vi "Inverse Kinematics.vi"(4 "Side":T2, 6 "Tolerance":dbl=0.1, 9 "Start":dbl[](array[numeric])=[0.0, -45.0, 0.0, 45.0, 0.0, 90.0, 0.0] format="%.3f", 10 "Goal-matrix":T1 format="%.3f", 11 "Label":string) -> (0 "Found":bool, 1 "Error":dbl, 2 "J":dbl[](array[numeric]) format="%.3f", 3 "Label":string)   [LabVIEW 2013]
uses:
  <vilib>/Analysis/Matrix/Datatypes/RealMatrix.ctl
  ROS/Code/SubVIs/BaxterSide.ctl
  <vilib>/Analysis/baseanly.llb/Real A x B.vi
  Fwd Kenimatics - array.vi
  <vilib>/Analysis/baseanly.llb/Real Inverse Matrix.vi
  Arm Globals.vi
  <vilib>/Analysis/NI_AALBase.lvlib
  <vilib>/Analysis/Matrix/NI_Matrix.lvlib
panel:
  in  "Joints":dbl[](array[numeric])=[0.0, 0.0, 0.0, 0.0, 0.0, -0.0, 0.0]
  out "Matrix":T1 format="%.3f"
  out "A x B":T1 format="%.3f"
  out "appended array":dbl[](array[numeric]) format="%.1f"
  out "Error History":dbl[](array[numeric])
  out "step":dbl format="%.6f"
  out "Count":i32
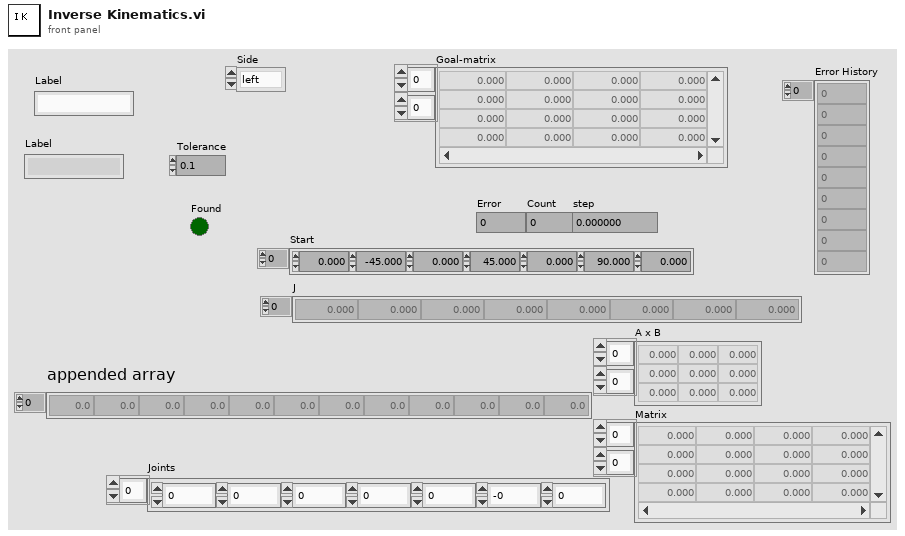
[diagram p1: front panel]
types:
  T1 = typedef "NI_Matrix.lvlib/RealMatrix.ctl" = dbl[][]
  T2 = typedef "BaxterSide.ctl" = enum16{"left", "right"}
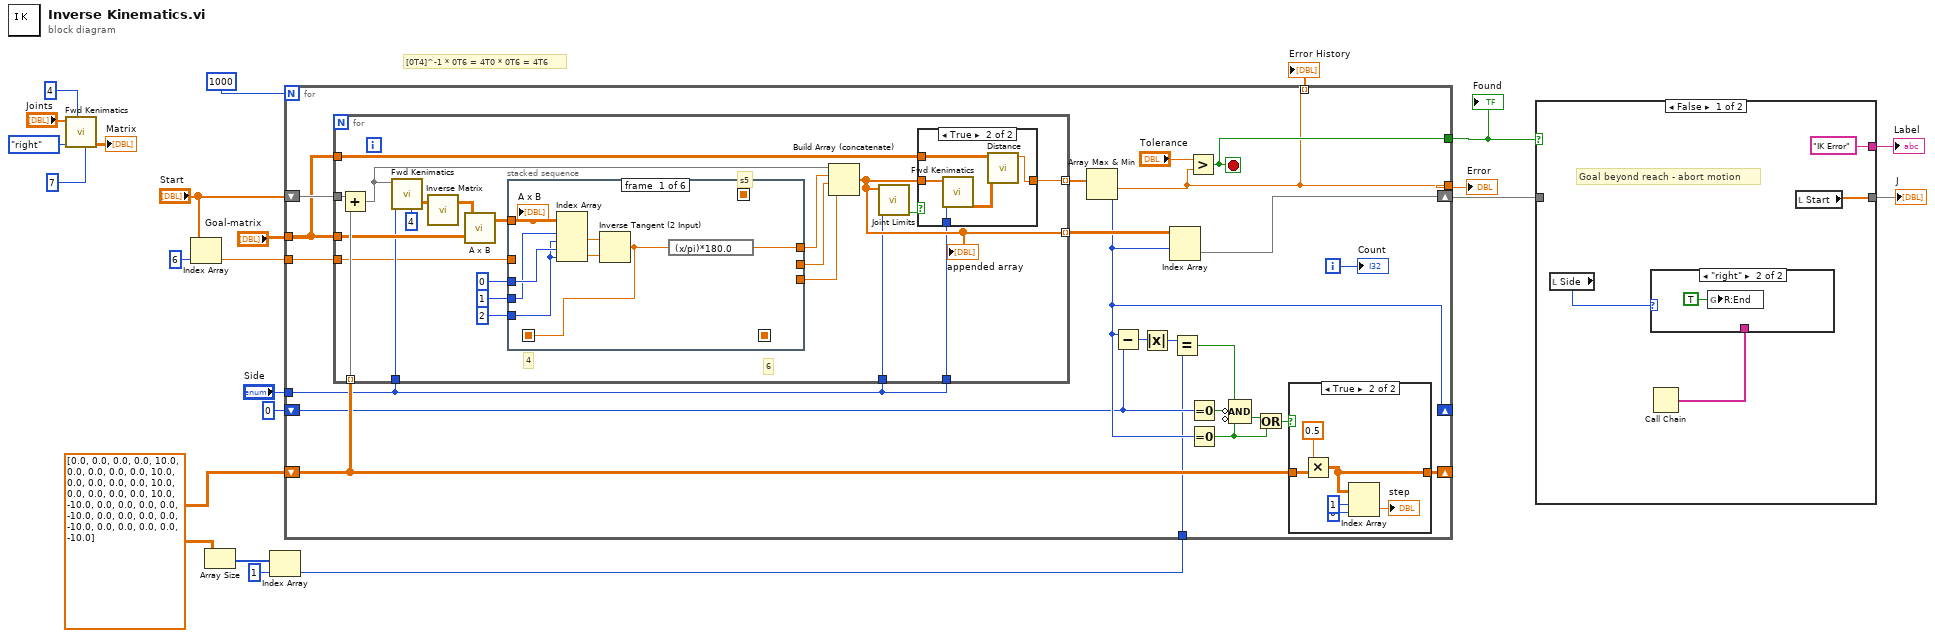
[diagram p0: block diagram]
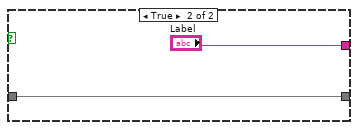
[diagram p3: hidden frame]
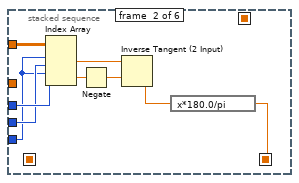
[diagram p5: hidden frame]
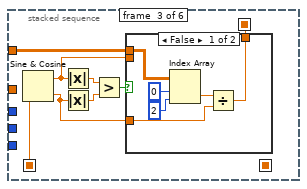
[diagram p6: hidden frame]
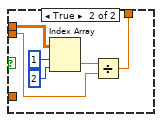
[diagram p7: hidden frame]
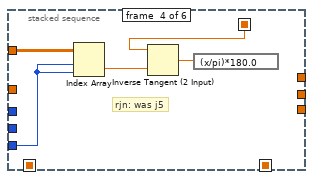
[diagram p8: hidden frame]
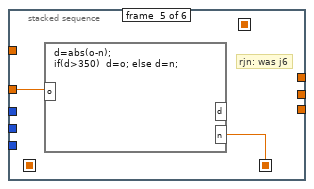
[diagram p9: hidden frame]
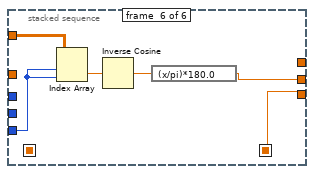
[diagram p10: hidden frame]
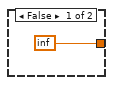
[diagram p11: hidden frame]
diagram:
  w16 = dbl[][] [[0.0, 0.0, 0.0, 0.0], [10.0, 0.0, 0.0, 0.0], [0.0, 10.0, 0.0, 0.0], [0.0, 0.0, 10.0, 0.0], [0.0, 0.0, 0.0, 10.0], [-10.0, 0.0, 0.0, 0.0], [0.0, -10.0, 0.0, 0.0], [0.0, 0.0, -10.0, 0.0], [0.0, 0.0, 0.0, -10.0]]
  # "[0T4]^-1 * 0T6 = 4T0 * 0T6 = 4T6"
  n1 = call-poly "Fwd Kenimatics.vi"("To"=7, "From"=4, "Side"=BaxterSide."right", "Joints"="Joints") -> ("Matrix"=→"Matrix":T1)  [unwired: 6 in, 1 out]
  n2 = Index Array(array="Start", index=6) -> (element=w9:dbl)
  n3 = Array Size(array=w16) -> (size(s)=w19:i32[])
  n4 = Index Array(array=w19, index=1) -> (element=w17:i32)
  n5 = for {
    N: 1000 -> [_]
    shift-right: [w43] -> w13
    shift-left: "Start" -> [w30]
    tunnel: [w24] -> w22
    shift-right: [w41] -> _
    shift-left: w16 -> [w40]
    shift-right: [w39] -> _
    shift-left: 0 -> [w32]
    tunnel: "Goal-matrix" -> [w26]
    tunnel: w17 -> [w29]
    tunnel: [w28] -> w8
    tunnel: "Side" -> [w25]
    tunnel: [w24] -> w14 mode=indexing
    tunnel: w9 -> [w23]
    i -> [w42]
    stop <- w28 stop-if-true
    n6 = for {
      tunnel: w40 -> [w70] mode=indexing
      tunnel: [w73] -> w45 mode=indexing
      tunnel: [w68] -> w44 mode=indexing
      tunnel: w30 -> [w71]
      tunnel: w26 -> [w69]
      tunnel: w26 -> [w60]
      tunnel: w25 -> [w56]
      tunnel: w25 -> [w55]
      tunnel: w25 -> [w54]
      tunnel: w23 -> [w53]
      # "6"
      # "s5"
      # "4"
      n7 = Add(x=w71, y=w70) -> (x+y=w57:dbl[])
      n8 = call-poly "Fwd Kenimatics.vi"("To"=4 ("# of Angles"), "Side"=w56, "Joints"=w57) -> ("Matrix"=w58:T1)  [unwired: 7 in, 1 out]
      n9 = call-poly <vilib>:"Inverse Matrix.vi"("Input Matrix"=w58) -> ("Inverse Matrix"=w67:T1)  [unwired: 1 in, 1 out]
      n10 = call-poly <vilib>:"A x B.vi"("B"=w69, "A"=w67) -> ("A x B"=w66:T1)  [unwired: 1 out]
      n11 = stacked-sequence {
        seq-local: [w78 _ _ _ _ _] -> [_ _ w99 _ _ _]
        seq-local: [_ _ w92 _ _ _] -> [_ _ _ w113 _ _]
        seq-local: [_ w83 _ _ _ _] -> [_ _ _ _ w118 w119]
        tunnel: [_ _ _ _ _ w119] -> w64
        tunnel: [w79 _ _ _ _ _] -> w72
        tunnel: w66 -> [w80 w90 w93 w116 _ w124]
        tunnel: [_ _ _ _ _ w120] -> w65
        tunnel: 0 ("index (col)") -> [w77 w86 _ _ _ _]
        tunnel: 1 ("index (row)") -> [w76 w85 _ _ _ _]
        tunnel: 2 ("index (row)") -> [w75 w84 _ w115 _ w123]
        tunnel: w53 -> [_ _ _ _ w117 _]
        frame #0 {
          n12 = Index Array(array=w80, index (row) #1=w76, index (col) #1=w75, index (row) #2=w77, index (col) #2=w75) -> (element #1=w81:dbl, element #2=w82:dbl)
          n13 = Inverse Tangent (2 Input)(1:w82, 2:w81) -> (0:w78:dbl)
          n14 = expression code="(x/pi)*180.0" ("radians to degrees")(w78) -> (w79:dbl)
          "A x B" <- w80
        }
        frame #1 {
          n15 = Index Array(array=w90, index (row) #1=w84, index (col) #1=w85, index (row) #2=w84, index (col) #2=w86) -> (element #1=w91:dbl, element #2=w89:dbl)
          n16 = Negate(x=w89) -> (-x=w88:dbl)
          n17 = Inverse Tangent (2 Input)(1:w88, 2:w91) -> (0:w87:dbl)
          n18 = expression code="x*180.0/pi" ("radians to degrees")(w87) -> (w83:dbl)
        }
        frame #2 {
          n19 = Sine & Cosine(0:w99) -> (1:w95:dbl, 2:w94:dbl)
          n20 = Absolute Value(x=w95) -> (abs(x)=w98:dbl)
          n21 = Absolute Value(x=w94) -> (abs(x)=w97:dbl)
          n22 = Greater?(x=w98, y=w97) -> (0:w96:bool)
          n23 = case shown="False" w96 {
            tunnel: w95 -> [_ w107]
            tunnel: w94 -> [w101 _]
            tunnel: w93 -> [w102 w111]
            tunnel: [w100 w106] -> w92
            frame False {
              n24 = Index Array(array=w102, index (row)=0, index (col)=2 ("disabled index (col)")) -> (element=w105:dbl)
              n25 = Divide(x=w105, y=w101) -> (x/y=w100:dbl)
            }
            frame True {
              n26 = Index Array(array=w111, index (row)=1, index (col)=2 ("disabled index (col)")) -> (element=w108:dbl)
              n27 = Divide(x=w108, y=w107) -> (x/y=w106:dbl)
            }
          }
        }
        frame #3 {
          # "rjn: was j5"
          n28 = Index Array(array=w116, index (row)=w115, index (col)=w115) -> (element=w114:dbl)
          n29 = Inverse Tangent (2 Input)(1:w114, 2:w113) -> (0:w112:dbl)
          n30 = expression code="(x/pi)*180.0" ("radians to degrees")(w112) -> ()  [unwired: 1 out]
        }
        frame #4 {
          # "rjn: was j6"
          n31 = formula code="d=abs(o-n);\nif(d>350)  d=o; else d=n;"("o"=w117, "n"=w118) -> ()  [unwired: 1 out]
        }
        frame #5 {
          n32 = Index Array(array=w124, index (row)=w123, index (col)=w123) -> (element=w122:dbl)
          n33 = Inverse Cosine(1:w122) -> (0:w121:dbl)
          n34 = expression code="(x/pi)*180.0" ("radians to degrees")(w121) -> (w120:dbl)
        }
      }
      n35 = Build Array (concatenate)(w57, w72, w65, w64) -> (w68:dbl[])
      "appended array" <- w68
      n36 = call "Joint Limits.vi"("Side"=w54, "Joints"=w68) -> ("In Range"=w74:bool)  [unwired: 9 in]
      n37 = case shown="True" w74 {
        tunnel: w68 -> [_ w130]
        tunnel: [inf w126] -> w73
        tunnel: w60 -> [_ w129]
        tunnel: w55 -> [_ w128]
        frame False {
        }
        frame True {
          n38 = call-poly "Fwd Kenimatics.vi"("Side"=w128, "Joints"=w130) -> ("Matrix"=w127:T1)  [unwired: 8 in, 1 out]
          n39 = call "Distance.vi"("Pose 2"=w127, "Pose 1"=w129) -> ("Distance"=w126:dbl)  [unwired: 9 in]
        }
      }
    }
    n40 = Array Max & Min(array=w45) -> (min value=w24:dbl, min index (indices)=w39:i32)  [unwired: 2 out]
    n41 = Subtract(x=w39, y=w32) -> (x-y=w38:i32)
    n42 = Absolute Value(x=w38) -> (abs(x)=w37:i32)
    n43 = Index Array(array=w44, index (row)=w39) -> (element=w43:dbl[])  [unwired: 1 in]
    n44 = Equal?(x=w37, y=w29) -> (x = y?=w34:bool)
    n45 = Greater?(x="Tolerance", y=w24) -> (0:w28:bool)
    n46 = Equal To 0?(x=w32) -> (x = 0?=w31:bool)
    n47 = Equal To 0?(x=w39) -> (x = 0?=w33:bool)
    n48 = Compound Arithmetic op=AND(w34, invert w31, invert w33) -> (w36:bool)
    n49 = Or(x=w36, y=w33) -> (x .or. y?=w35:bool)
    n50 = case shown="True" w35 {
      tunnel: w40 -> [w46 w52]
      tunnel: [w46 w50] -> w41
      frame False {
      }
      frame True {
        n51 = Multiply(x=0.5, y=w52) -> (x*y=w50:dbl[][])
        n52 = Index Array(array=w50, index (row)=1, index (col)=0 ("disabled index (col)")) -> (element=→"step":dbl)
      }
    }
    "Count" <- w42
  }
  "Error" <- w22
  "Found" <- w8
  "Error History" <- w14
  n53 = case shown="False" w8 {
    tunnel: w13 -> [_ w137]
    tunnel: [w134 w137] -> w7
    tunnel: ["IK Error" ("Label") "Label"] -> w6
    frame False {
      # "Goal beyond reach - abort motion"
      n54 = local read "Side"() -> (w132:T2)
      n55 = Call Chain() -> (call chain=w131:string[])
      n56 = case shown="\"right\"" w132 {
        tunnel: w131 -> [_ _]
        frame "left", Default {
        }
        frame "right" {
          n57 = global write "Arm Globals.vi" "R:End"(TRUE ("R:End")) -> ()
        }
      }
      n58 = local read "Start"() -> (w134:dbl[])
    }
    frame True {
    }
  }
  "J" <- w7
  "Label" <- w6
